vi "PH_Names.concatenate Names.vi"(1 "Communication Type (no info)":T1, 2 "Devices (no info)":T4, 3 "PU (no info)":T3, 4 "Subsystem":T2) -> (0 "Subsystem_PU_Devices_Comm Type":string)   [LabVIEW 2014, in "PH_Common.lvlib"]
doc: "This VI concatenates, depending from the connected inputs, a string. Subsystem must be connected; if this is \"no info\", N/A is given out. If one or all ao the other inputs are \"no info\" (what is default), the part of the string is not concatenated. Seperator is a underline \"_\"."
uses:
  PH_Common.lvlib
  PH_PP_Common/PH_PP_Common.Devices.ctl
  PH_PP_Common/PH_PP_Common.PUs.ctl
  PH_Names.Subsystems.ctl
  PH_Names.Communication Type.ctl
  PH_PP_Common/PH_PP_Common.lvlib
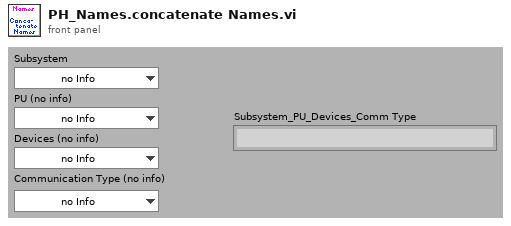
[diagram p1: front panel]
types:
  T1 = typedef "PH_Common.lvlib/PH_Names.Communication Type.ctl" = enum16{"no Info", "SE", "SA", "AE", "AA", "DE", "DA", "DIM"}
  T2 = typedef "PH_Common.lvlib/PH_Names.Subsystems.ctl" = enum16{"no Info", "fs-FE", "ns-FE", "PA", "MA", "MAS", "COS", "Exp-LB", "Exp-LL", "PP", "PILS"}
  T3 = typedef "PH_PP_Common.lvlib/PH_PP_Common.PUs.ctl" = enum16{"no Info", "PA-19mm-1", "PA-19mm-2", "PA-45mm-PILC", "PA-45mm-MAIN", "MA-PU-1", "MA-PU-2", "MA-PU-3", "MA-PU-4", "MA-PU-5", "MA-PU-6", "MA-FR", "MA-PILC", "PA-45mm-DP"}
  T4 = typedef "PH_PP_Common.lvlib/PH_PP_Common.Devices.ctl" = enum16{"no Info", "Igni", "RR", "DumpRoss", "PSU", "Trigger", "HV-Meas", "Rods", "Chiller", "Conductivity", "Mercury"}
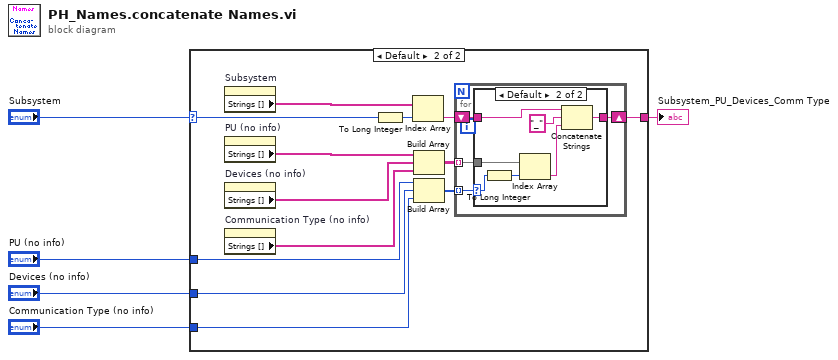
[diagram p0: block diagram]
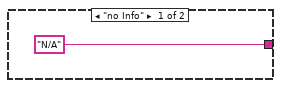
[diagram p2: hidden frame]
diagram:
  n1 = case shown="Default" "Subsystem" {
    selector: "Subsystem" -> [_ w7]
    tunnel: "Devices (no info)" -> [_ w19]
    tunnel: "PU (no info)" -> [_ w18]
    tunnel: "Communication Type (no info)" -> [_ w15]
    tunnel: ["N/A" w13] -> w2
    frame "no Info" {
    }
    frame Default {
      n2 = property on="Subsystem" class="Enum (strict)"() -> ("Strings []"=w9:string[])  [unwired: 2 in, 2 out]
      n3 = property on="PU (no info)" class="Enum (strict)"() -> ("Strings []"=w17:string[])  [unwired: 2 in, 2 out]
      n4 = property on="Devices (no info)" class="Enum (strict)"() -> ("Strings []"=w16:string[])  [unwired: 2 in, 2 out]
      n5 = property on="Communication Type (no info)" class="Enum (strict)"() -> ("Strings []"=w14:string[])  [unwired: 2 in, 2 out]
      n6 = To Long Integer(number=w7) -> (32bit integer=w10:i32)
      n7 = Index Array(array=w9, index=w10) -> (element=w8:string)
      n8 = Build Array(w17, w16, w14) -> (w12:string[][])
      n9 = Build Array(w18, w19, w15) -> (w11:u16[])
      n10 = for {
        shift-right: [w23] -> w13
        shift-left: w8 -> [w22]
        tunnel: w12 -> [w21] mode=indexing
        tunnel: w11 -> [w20] mode=indexing
        n11 = case shown="Default" w20 {
          selector: w20 -> [_ w25]
          tunnel: [w24 w31] -> w23
          tunnel: w22 -> [w24 w30]
          tunnel: w21 -> [_ w29]
          frame 0 {
          }
          frame Default {
            n12 = To Long Integer(number=w25) -> (32bit integer=w28:i32)
            n13 = Index Array(array=w29, index=w28) -> (element=w27:string)
            n14 = Concatenate Strings(w30, "_" ("string"), w27) -> (w31:string)
          }
        }
      }
    }
  }
  "Subsystem_PU_Devices_Comm Type" <- w2
